vi "CMD_ROTATETO.vi"(6 "Gantry in":refnum<class "Gantry.lvclass">, 8 "error in (no error)":errorcluster, 10 "Arguments":string[](array[string]), 11 "gScript Interpreter in":refnum<class "gScript Interpreter.lvclass">) -> (0 "error out":errorcluster, 3 "gScript Interpreter out":refnum<class "gScript Interpreter.lvclass">, 4 "Gantry out":refnum<class "Gantry.lvclass">)   [LabVIEW 2017, in "gScript Interpreter.lvclass"]
uses:
  gScript Interpreter.lvclass
  Shared Components/Gantry Class/Gantry.lvclass
  Shared Components/Orient3d Class/Orient3d.lvclass
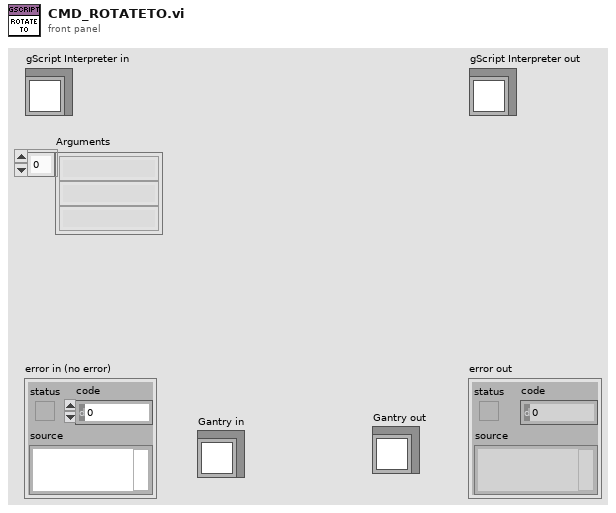
[diagram p1: front panel]
types:
  T1 = typedef "Memory Cell.ctl" = cluster{"type":T2, "x":dbl, "y":dbl, "z":dbl, "w":dbl}
  T2 = typedef "Memory Cell Type Enum.ctl" = enum16{"integer", "float", "vector", "rotation"}
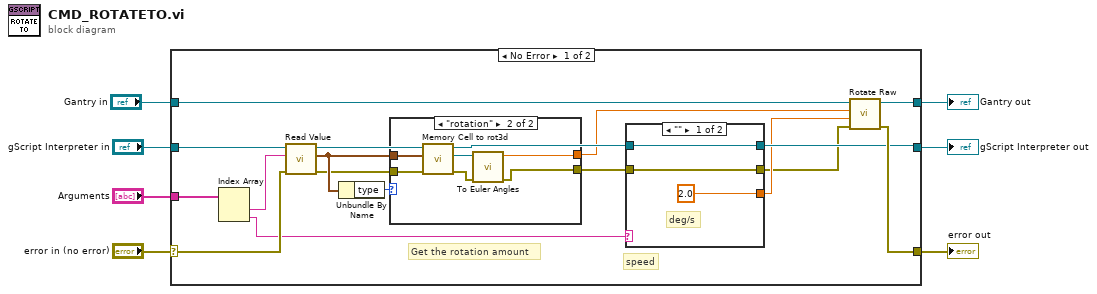
[diagram p0: block diagram]
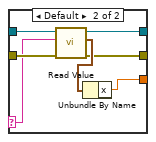
[diagram p2: hidden frame]
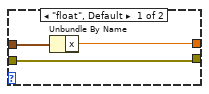
[diagram p3: hidden frame]
diagram:
  n1 = case shown="No Error" "error in (no error)" {
    selector: "error in (no error)" -> [w19 w45]
    tunnel: [w18 w45] -> w6
    tunnel: [w13 w44] -> w4
    tunnel: "gScript Interpreter in" -> [w22 w44]
    tunnel: "Arguments" -> [w21 _]
    tunnel: "Gantry in" -> [w24 w43]
    tunnel: [w23 w43] -> w1
    frame No Error {
      # "speed"
      # "Get the rotation amount"
      n2 = Index Array(array=w21) -> (element #1=w20:string, element #2=w15:string)  [unwired: 2 in]
      n3 = call-dynamic "Read Value.vi"("error in (no error)"=w19, "String in"=w20, "gScript Interpreter in"=w22) -> ("error out"=w12:errorcluster, "Memory Cell"=w16:T1, "gScript Interpreter out"=w14:refnum<class "gScript Interpreter.lvclass">)  [unwired: 6 in]
      n4 = Unbundle By Name(w16) -> ("type"=w17:T2)
      n5 = case shown="\"rotation\"" w17 {
        tunnel: w16 -> [w37 w42]
        tunnel: [w36 w40] -> w10
        tunnel: w12 -> [w35 w39]
        tunnel: [w35 w38] -> w11
        frame "float", Default {
          n6 = Unbundle By Name(w37) -> ("x"=w36:dbl)
        }
        frame "rotation" {
          n7 = call "Memory Cell to rot3d.vi"("Memory Cell"=w42) -> ("Orient3d out"=w41:refnum<class "Orient3d.lvclass">)  [unwired: 10 in]
          n8 = call "To Euler Angles.vi"("error in"=w39, "Orient3d in"=w41) -> ("error out"=w38:errorcluster, "psi/yaw"=w40:dbl)  [unwired: 6 in, 2 out]
        }
      }
      n9 = case shown="\"\"" w15 {
        selector: w15 -> [_ w31]
        tunnel: w14 -> [w27 w34]
        tunnel: w11 -> [w26 w33]
        tunnel: [w27 w32] -> w13
        tunnel: [w26 w29] -> w8
        tunnel: [2.0 w28] -> w9
        frame "" {
          # "deg/s"
        }
        frame Default {
          n10 = call-dynamic "Read Value.vi"("error in (no error)"=w33, "String in"=w31, "gScript Interpreter in"=w34) -> ("error out"=w29:errorcluster, "Memory Cell"=w30:T1, "gScript Interpreter out"=w32:refnum<class "gScript Interpreter.lvclass">)  [unwired: 6 in]
          n11 = Unbundle By Name(w30) -> ("x"=w28:dbl)
        }
      }
      n12 = call-dynamic "Rotate Raw.vi"("error in"=w8, "speed(deg/s)"=w9, "position(deg)"=w10, "Gantry in"=w24) -> ("error out"=w18:errorcluster, "Gantry out"=w23:refnum<class "Gantry.lvclass">)  [unwired: 6 in]
    }
    frame Error {
    }
  }
  "error out" <- w6
  "gScript Interpreter out" <- w4
  "Gantry out" <- w1
